vi "初始化SIEMENS.vi"(8 "错误输入（无错误）":errorcluster) -> (0 "错误输出":errorcluster, 2 "通讯状态":bool, 3 "gInitialSIEMENSS7":refnum<k24>)   [LabVIEW 2017]
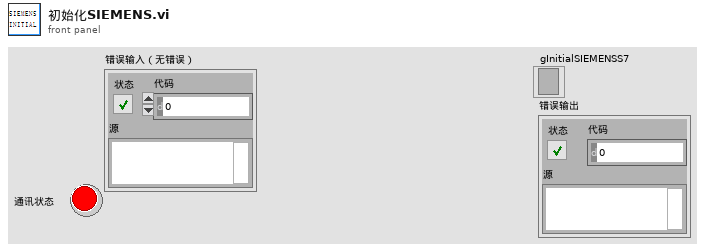
[diagram p1: front panel]
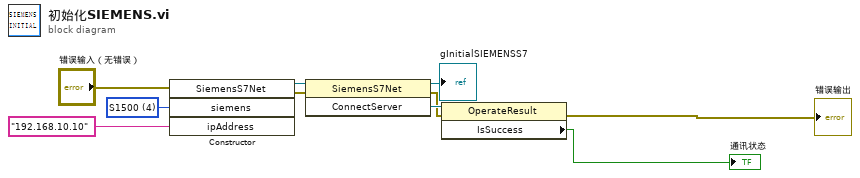
[diagram p0: block diagram]
diagram:
  w9 = 4 items=["S1200"=1, "S300"=2, "S400"=3, "S1500"=4, "S200Smart"=5] ("siemens")
  n1 = constructor class="SiemensS7Net"(error in="错误输入（无错误）", "siemens"=w9, "ipAddress"="192.168.10.10") -> (reference out=w7:refnum<k24>, error out=w6:errorcluster)  [unwired: 2 in, 3 out]
  n2 = invoke class="SiemensS7Net" method="ConnectServer"(reference=w7, error in=w6) -> (reference out=→"gInitialSIEMENSS7":refnum<k24>, error out=w2:errorcluster, "ConnectServer"=w10:refnum<k24>)  [unwired: 1 in]
  n3 = property class="OperateResult"(reference=w10, error in=w2) -> (error out=→"错误输出":errorcluster, "IsSuccess"=→"通讯状态":bool)  [unwired: 1 out]
